vi "Use a Filter Bank to Extract Signals.vi"() -> ()   [LabVIEW 2023]
doc: "This example demonstrates how to use a 2-band filter bank to extract the low frequency or high frequency signal from a combined signal.\n\nComplete the following steps to use this VI:\n1) Run this VI.\n2) The combined signal is two sine signals, which are specified by <b>Low Frequency</b> and <b>High Frequency</b>.\n3) In the <b>Extract High/Low?</b> box, select whether to extract the low frequency or high frequency sine signal."
uses:
  <vilib>/addons/Digital Filter Design/FilterBank.llb/Process/DFD 2-Band Filter Bank Decomposition (Wfm).vi
  <vilib>/addons/Digital Filter Design/FilterBank.llb/Process/DFD 2-Band Filter Bank Reconstruction (Wfm).vi
  <vilib>/measure/NI_MABase.lvlib
  <vilib>/addons/Digital Filter Design/NI_DigFilter_FilterBank.lvlib
panel:
  in  "Extract High/Low?":enum16{"Low Frequency", "High Frequency"}(ring)
  in  "stop":bool
  in  "High Frequency":dbl(knob)=317.0527598110056 scale=300.0..400.0
  in  "Low Frequency":dbl(knob)=22.556811219530754 scale=10.0..110.0
  out "Extracted Signal":waveform(dbl)(graph)
  out "Combined Signal":waveform(dbl)(graph)
  # "Select Help>>Show Context Help and move the cursor over the VI icon for more information."
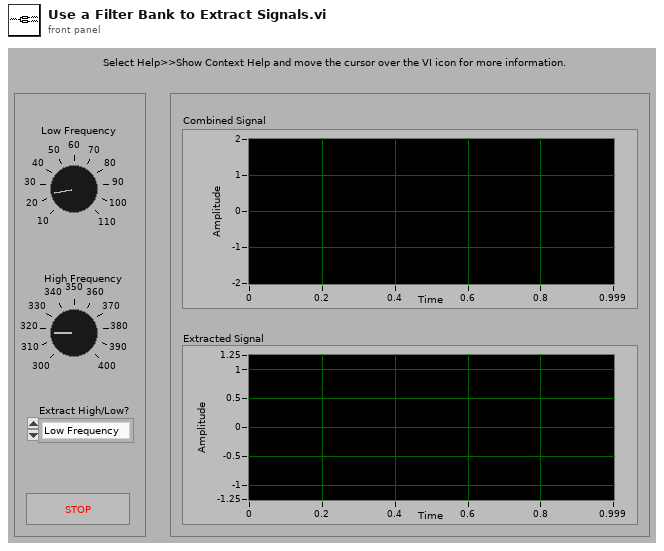
[diagram p1: front panel]
types:
  T1 = typedef "NI_DigFilter_FilterBank.lvlib/DFD Filter Bank Obj.ctl" = cluster{"mFBank_AnalysisFilters":T2[], "mFBank_SynthesisFilters":T2[], "mFBank_#Bands":i32, "mFBank_ProcMethod":T7, "mFBank_Coeffs":dbl[], "mFBank_Gain":dbl, "mFBank_Delay":i32, "mFBank_Type":T8}
  T2 = typedef "NI_DigFilterLicensed.lvlib/DFD Multirate Filter Obj.ctl" = cluster{"mMRate_Structure":enum16{"CIC", "FIR", "IIR", "Lattice"}, "mMRate_Mode":T3, "mMRate_Factor":i32, "mMRate_FIRParams":cluster{"mMRate_FIR_H":dbl[], "mMRate_FIR_IsNyquist?":bool, "mMRate_FIR_IsSymmetric?":bool}, "mMRate_CICParams":cluster{"mMRate_CIC_#Stage":i32, "mMRate_CIC_Lag":i32, "mMRate_CIC_Type":enum16{"Lowpass", "Highpass"}}, "mMRate_Order":i32, "mMRate_Version":string, "mMRate_Comments":string, "mMRate_RationalFactor":cluster{"mMRate_L":i32, "mMRate_M":i32}, "mMRate_Fs":dbl, "mMRate_Quantized?":bool, "mMRate_QFilterGain":dbl, "mMRate_CoefWl":i16, "mMRate_Scaling":cluster{"mMRate_ScaleByPowerOf2?":bool, "mMRate_ScaleType":T4}, "mMRate_InputWl":i16, "mMRate_OutputWl":i16, "mMRate_OutputMode":T5, "mMRate_MultMode":T6, "mMRate_BitPruning":bool, "mMRate_GainWl":i16, "mMRate_OutputFwl":i16, "mMRate_SumIwl":i16, "mMRate_InputIwl ":i16, "mMRate_SumWl":i16, "mMRate_CoefIwl":i16}
  T3 = typedef "NI_DigFilterLicensed.lvlib/DFD Multirate Mode.ctl" = i16
  T4 = typedef "NI_DigFilterLicensed.lvlib/DFD Coef Norm Type.ctl" = enum16{"No Norm", "Time Domain 1-Norm", "Time Domain 2-Norm", "Time Domain Inf-Norm"}
  T5 = typedef "NI_DigFilterLicensed.lvlib/DFD Round-off Mode.ctl" = enum16{"Nearest", "Truncation"}
  T6 = typedef "NI_DigFilterLicensed.lvlib/DFD FXP MRate Multiply Mode.ctl" = enum16{"Truncated", "Full"}
  T7 = typedef "NI_DigFilter_FilterBank.lvlib/DFD Filter Bank Processing Method.ctl" = enum16{"General", "2-Band QMF Lattice", "Cosine-Modulated"}
  T8 = typedef "NI_DigFilter_FilterBank.lvlib/DFD Filter Bank Type.ctl" = u16
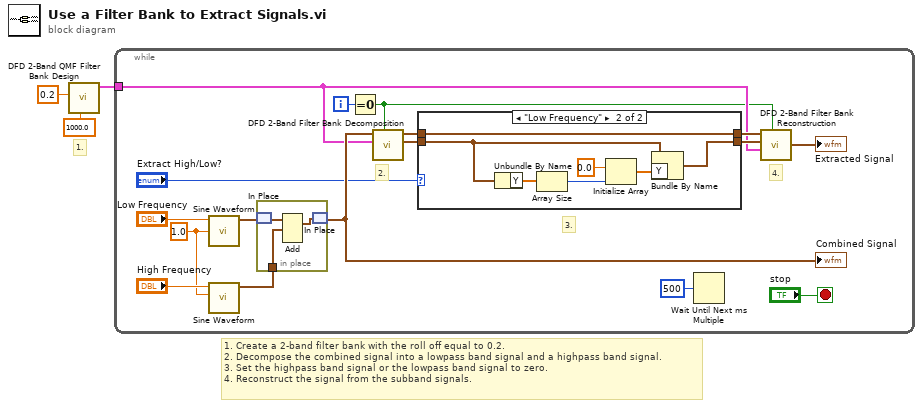
[diagram p0: block diagram]
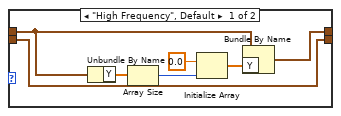
[diagram p2: hidden frame]
diagram:
  # "1."
  # "1. Create a 2-band filter bank with the roll off equal to 0.2.\n2. Decompose the combined signal into a lowpass band signal and a highpass band signal.\n3. Set the highpass band signal or the lowpass band signal to zero.\n4. Reconstruct the signal from the subband signals."
  n1 = call <vilib>:"DFD 2-Band QMF Filter Bank Design.vi"("fs in [Hz]"=1000.0, "roll off"=0.2) -> ("filter bank out"=w3:T1)  [unwired: 7 in, 2 out]
  n2 = while {
    tunnel: w3 -> [w8]
    i -> [w7]
    stop <- "stop" stop-if-true
    w5 = 1.0 ("amplitude")
    # "4."
    # "3."
    # "2."
    n3 = call <vilib>:"Sine Waveform.vi"("amplitude"=w5, "frequency"="Low Frequency") -> ("signal out"=w18:waveform(dbl))  [unwired: 8 in, 1 out]
    n4 = call <vilib>:"Sine Waveform.vi"("amplitude"=w5, "frequency"="High Frequency") -> ("signal out"=w17:waveform(dbl))  [unwired: 8 in, 1 out]
    n5 = in-place {
      in-place-border: w17 -> [w22]
      n6 = in-place-match #1(w18) -> (w23:waveform(dbl))
      n7 = Add(1:w22, 2:w23) -> (0:w21:waveform(dbl))  [unwired: 1 in, 1 out]
      n8 = in-place-match #1(w21) -> (w11:waveform(dbl))
    }
    "Combined Signal" <- w11
    n9 = Equal To 0?(x=w7) -> (x = 0?=w6:bool)
    n10 = call-poly <vilib>:"DFD 2-Band Filter Bank Decomposition.vi"("init? (F)"=w6, "filter bank in"=w8, "signal in"=w11) -> ("highpass band"=w15:waveform(dbl), "lowpass band"=w13:waveform(dbl))  [unwired: 6 in, 1 out]
    n11 = case shown="\"Low Frequency\"" "Extract High/Low?" {
      tunnel: w15 -> [w24 w33]
      tunnel: [w26 w31] -> w10
      tunnel: w13 -> [w25 w31]
      tunnel: [w24 w32] -> w9
      frame "High Frequency", Default {
        n12 = Unbundle By Name(w25) -> ("Y"=w30:dbl[])
        n13 = Array Size(array=w30) -> (size(s)=w29:i32)
        n14 = Initialize Array(0.0 ("element"), w29) -> (w27:dbl[])
        n15 = Bundle By Name(cluster=w25, "Y"=w27) -> (w26:waveform(dbl))
      }
      frame "Low Frequency" {
        n16 = Unbundle By Name(w33) -> ("Y"=w37:dbl[])
        n17 = Array Size(array=w37) -> (size(s)=w36:i32)
        n18 = Initialize Array(0.0 ("element"), w36) -> (w34:dbl[])
        n19 = Bundle By Name(cluster=w33, "Y"=w34) -> (w32:waveform(dbl))
      }
    }
    n20 = Wait Until Next ms Multiple(millisecond multiple=u32 500) -> ()  [unwired: 1 out]
    n21 = call-poly <vilib>:"DFD 2-Band Filter Bank Reconstruction.vi"("init? (F)"=w6, "filter bank in"=w8, "highpass band"=w9, "lowpass band"=w10) -> ("signal out"=→"Extracted Signal":waveform(dbl))  [unwired: 6 in, 1 out]
  }
